vi "USB_DAQ__DS3231_RTC_Test_READ_WRITE_Date_Time.vi"() -> ()   [LabVIEW 2022 SP3]
doc: "Petrus Prins\n4 August 2026"
uses:
  DS3231_Date_Time.ctl
panel:
  out "Zero_Date_Time_OK":bool
  in  "Write_Zero_Date_Time_To_DS3231":bool
  out "Date_Time_Write_OK":bool
  in  "Write_PC_Date_Time_To_DS3231":bool
  in  "Read_PC_System_Date_Time":bool
  out "PC_Date_Time":T1
  out "DS3231_Date_Time":T1
  out "Deg.C":dbl format="%-2_6g"
  out "Temp_Data_Valid":bool
  in  "Read_DS3231_Temperature":bool
  out "Time_Data_Valid":bool
  out "Raw_RTC_Data":u8[](array[numeric]) format="%2x"
  in  "Read_DS3231_Date_Time":bool
  in  "DS3231.Addr":u8=104 format="%02x"
  in  "Stop":bool
  # "DS3231"
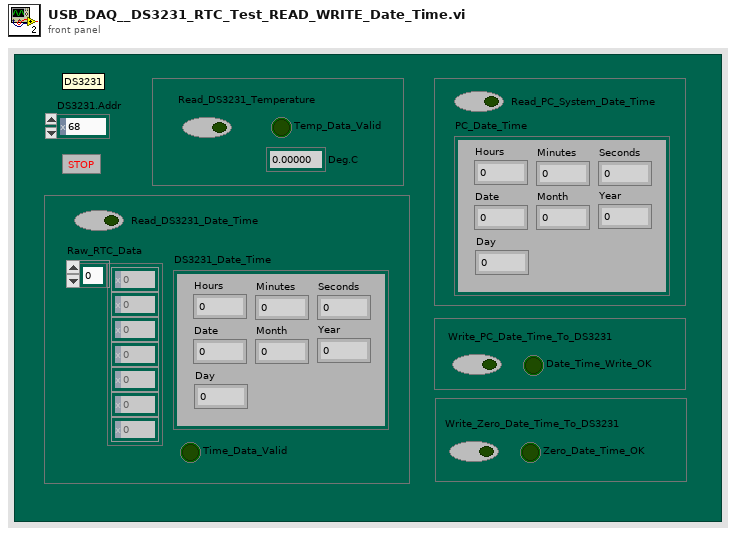
[diagram p1: front panel]
types:
  T1 = typedef "DS3231_Date_Time.ctl" = cluster{"Seconds":u8, "Minutes":u8, "Hours":u8, "Day":u8, "Date":u8, "Month":u8, "Year":u8}
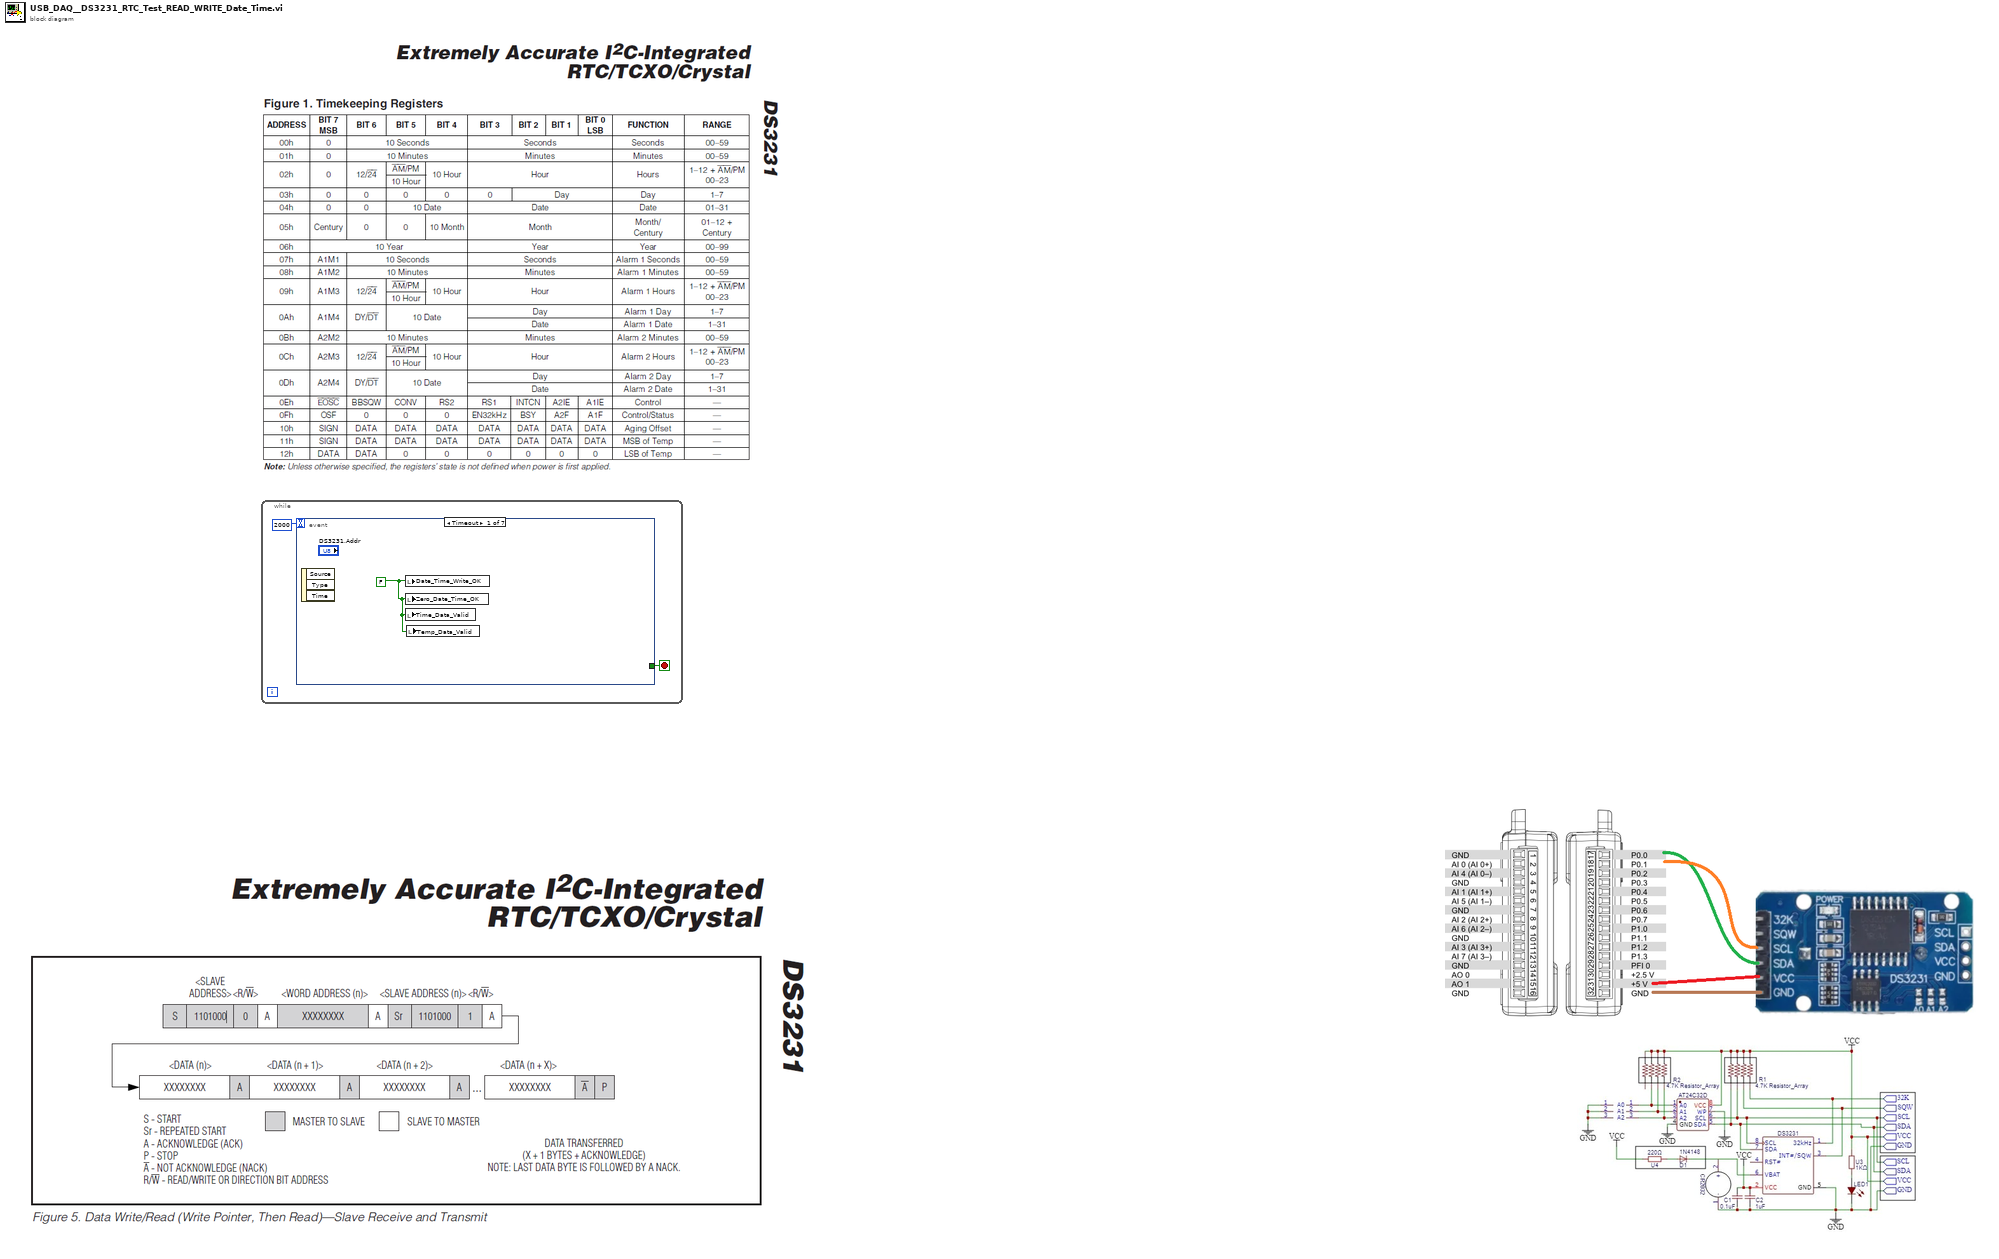
[diagram p0: block diagram]
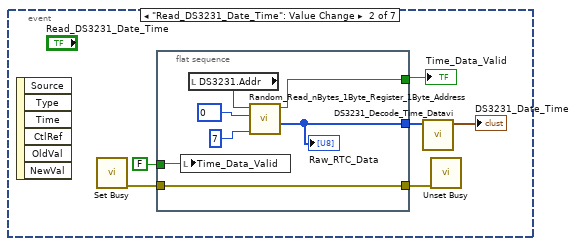
[diagram p2: hidden frame]
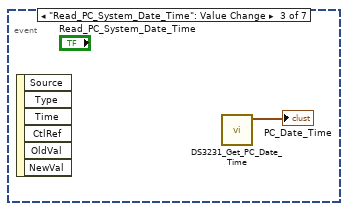
[diagram p3: hidden frame]
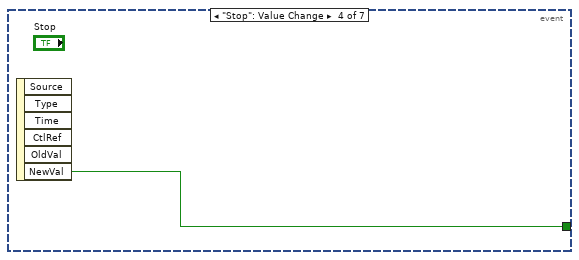
[diagram p4: hidden frame]
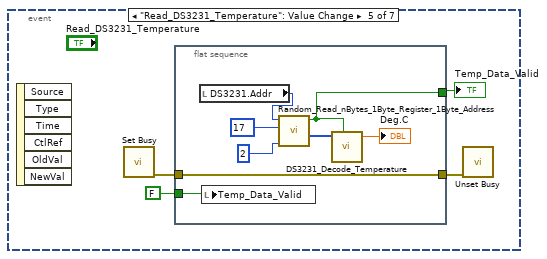
[diagram p5: hidden frame]
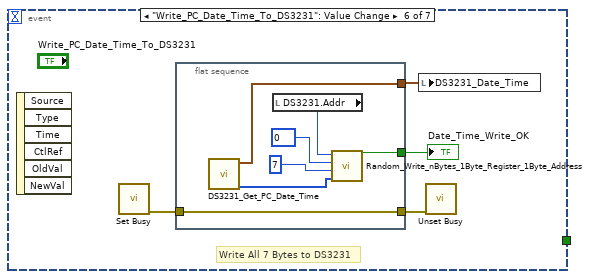
[diagram p6: hidden frame]
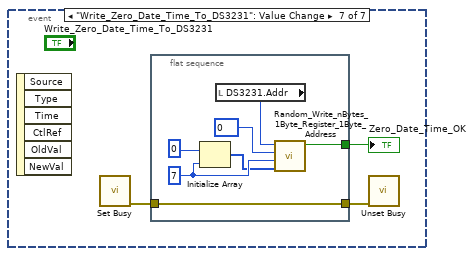
[diagram p7: hidden frame]
diagram:
  n1 = while {
    stop <- w1 stop-if-true
    n2 = event shown="[0] Timeout" {
      selector: _ -> [_ _ _ _ _ _ _]
      dyn-events: _ -> [_ _ _ _ _ _ _]
      timeout: 2000 -> [_ _ _ _ _ _ _]
      tunnel: [_ _ _ w18 _ _ _] -> w1
      event Timeout {
        w3 = FALSE ("Date_Time_Write_OK")
        n3 = event-data() -> ()  [unwired: 1 in, 3 out]
        n4 = local write "Date_Time_Write_OK"(w3) -> ()
        n5 = local write "Zero_Date_Time_OK"(w3) -> ()
        n6 = local write "Time_Data_Valid"(w3) -> ()
        n7 = local write "Temp_Data_Valid"(w3) -> ()
      }
      event "Read_DS3231_Date_Time": Value Change {
        n8 = event-data() -> ()  [unwired: 1 in, 6 out]
        n9 = call <vilib>:"Set Busy.vi"() -> ("error out"=w9:errorcluster)  [unwired: 10 in, 1 out]
        n10 = flat-sequence {
          tunnel: w9 -> [w16]
          tunnel: [w16] -> w8
          tunnel: FALSE ("Data_Valid") -> [w15]
          tunnel: [w11] -> w5
          tunnel: [w10] -> w4
          frame #0 {
            n11 = local write "Time_Data_Valid"(w15) -> ()
            n12 = local read "DS3231.Addr"() -> (w14:u8)
            n13 = call "Random_Read_nBytes_1Byte_Register_1Byte_Address.vi"("Rx.Byte.Count.In"=7, "Register.Addr"=u8 0, "Device.Addr"=w14) -> ("Rx.Array.Out"=w11:u8[], "Data_Valid"=w10:bool)  [unwired: 4 in]
            "Raw_RTC_Data" <- w11
          }
        }
        n14 = call "DS3231_Decode_Time_Datavi.vi"("Raw_RTC_Data_In"=w5) -> ("DS3231_Date_Time"=→"DS3231_Date_Time":T1)  [unwired: 10 in]
        n15 = call <vilib>:"Unset Busy.vi"("error in (no error)"=w8) -> ()  [unwired: 10 in, 1 out]
        "Time_Data_Valid" <- w4
      }
      event "Read_PC_System_Date_Time": Value Change {
        n16 = event-data() -> ()  [unwired: 1 in, 6 out]
        n17 = call "DS3231_Get_PC_Date_Time.vi"() -> ("PC_Date_Time"=→"PC_Date_Time":T1)  [unwired: 10 in, 1 out]
      }
      event "Stop": Value Change {
        n18 = event-data() -> ("NewVal"=w18:bool)  [unwired: 1 in, 5 out]
      }
      event "Read_DS3231_Temperature": Value Change {
        n19 = event-data() -> ()  [unwired: 1 in, 6 out]
        n20 = call <vilib>:"Set Busy.vi"() -> ("error out"=w22:errorcluster)  [unwired: 10 in, 1 out]
        n21 = flat-sequence {
          tunnel: w22 -> [w29]
          tunnel: [w29] -> w21
          tunnel: FALSE ("Temp_Data_Valid") -> [w27]
          tunnel: [w23] -> w19
          frame #0 {
            n22 = local read "DS3231.Addr"() -> (w28:u8)
            n23 = local write "Temp_Data_Valid"(w27) -> ()
            n24 = call "Random_Read_nBytes_1Byte_Register_1Byte_Address.vi"("Rx.Byte.Count.In"=2, "Register.Addr"=u8 17, "Device.Addr"=w28) -> ("Rx.Array.Out"=w24:u8[], "Data_Valid"=w23:bool)  [unwired: 4 in]
            n25 = call "DS3231_Decode_Temperature.vi"("Data_Valid?"=w23, "DS3231.Temp_Data_In"=w24) -> ("Temp.DegC_Out"=→"Deg.C":dbl)  [unwired: 9 in]
          }
        }
        n26 = call <vilib>:"Unset Busy.vi"("error in (no error)"=w21) -> ()  [unwired: 10 in, 1 out]
        "Temp_Data_Valid" <- w19
      }
      event "Write_PC_Date_Time_To_DS3231": Value Change {
        # "Write All 7 Bytes to DS3231"
        n27 = event-data() -> ()  [unwired: 1 in, 6 out]
        n28 = call <vilib>:"Set Busy.vi"() -> ("error out"=w33:errorcluster)  [unwired: 10 in, 1 out]
        n29 = flat-sequence {
          tunnel: [w39] -> w34
          tunnel: [w38] -> w31
          tunnel: w33 -> [w37]
          tunnel: [w37] -> w32
          frame #0 {
            n30 = call "DS3231_Get_PC_Date_Time.vi"() -> ("DS3231_Friendly_Array"=w35:u8[], "PC_Date_Time"=w38:T1)  [unwired: 10 in]
            n31 = local read "DS3231.Addr"() -> (w41:u8)
            n32 = call "Random_Write_nBytes_1Byte_Register_1Byte_Address.vi"("Tx.Array.Out"=w35, "Tx.Byte.Count"=7, "Register.Addr"=u8 0, "Device.Addr"=w41) -> ("Data_Valid"=w39:bool)  [unwired: 4 in]
          }
        }
        n33 = local write "DS3231_Date_Time"(w31) -> ()
        n34 = call <vilib>:"Unset Busy.vi"("error in (no error)"=w32) -> ()  [unwired: 10 in, 1 out]
        "Date_Time_Write_OK" <- w34
      }
      event "Write_Zero_Date_Time_To_DS3231": Value Change {
        n35 = event-data() -> ()  [unwired: 1 in, 6 out]
        n36 = call <vilib>:"Set Busy.vi"() -> ("error out"=w44:errorcluster)  [unwired: 10 in, 1 out]
        n37 = flat-sequence {
          tunnel: [w49] -> w42
          tunnel: w44 -> [w48]
          tunnel: [w48] -> w43
          frame #0 {
            w46 = 7 ("Tx.Byte.Count")
            n38 = Initialize Array(u8 0 ("Tx.Byte.Count"), w46) -> (w45:u8[])
            n39 = local read "DS3231.Addr"() -> (w51:u8)
            n40 = call "Random_Write_nBytes_1Byte_Register_1Byte_Address.vi"("Tx.Array.Out"=w45, "Tx.Byte.Count"=w46, "Register.Addr"=u8 0, "Device.Addr"=w51) -> ("Data_Valid"=w49:bool)  [unwired: 4 in]
          }
        }
        n41 = call <vilib>:"Unset Busy.vi"("error in (no error)"=w43) -> ()  [unwired: 10 in, 1 out]
        "Zero_Date_Time_OK" <- w42
      }
    }
  }
